vi "Read.vi"(8 "error in (no error)":errorcluster, 11 "SMO.Instrument":refnum<class "SMO.InstrumentDriver.lvclass">) -> (0 "error out":errorcluster, 2 "value":T1, 3 "SMO.Instrument out":refnum<class "SMO.InstrumentDriver.lvclass">)   [LabVIEW 2013, in "SMO.InstrumentDriver.lvclass"]
doc: "---------------------------------------------------------------\nJKI State Machine Objects™\nhttp://jki.net/state-machine-objects/\nCopyright (C) 2005-2015, JKI <info@jki.net>\nALL RIGHTS RESERVEDJKI State Machine Objects (SMO) 1.0.0.5\nJKI - JKI\nCopyright (c) 2016, JKI"
uses:
  SMO.InstrumentDriver.lvclass
  Typedefs/ReadData.ctl
panel:
  # "For instructions on how to use the JKI State Machine Objects, examples and video tutorials, visit:\nhttp://jki.net/state-machine-objects/\n\nJKI State Machine Objects™\nhttp://jki.net/state-machine-objects/\nCopyright (C) 2005-2015, JKI <info@jki.net>\nALL RIGHTS RESERVED"
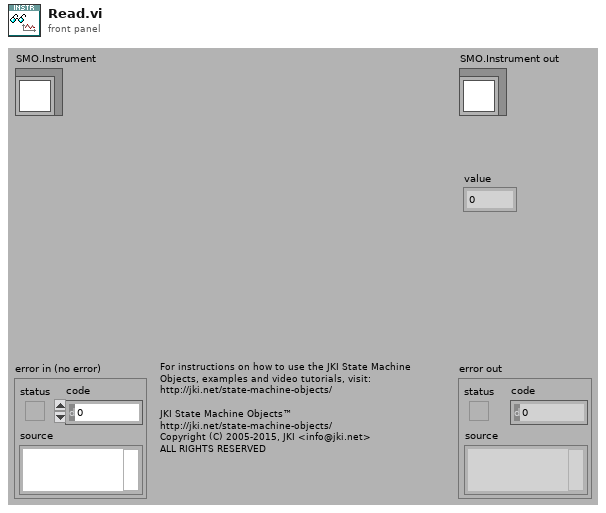
[diagram p1: front panel]
types:
  T1 = typedef "SMO.InstrumentDriver.lvclass/ReadData.ctl" = dbl
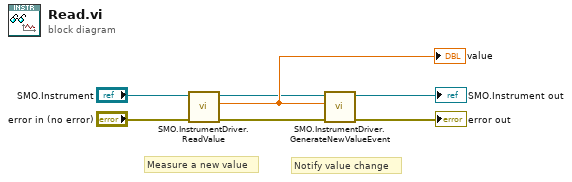
[diagram p0: block diagram]
diagram:
  # "Notify value change"
  # "Measure a new value"
  n1 = call-dynamic "SMO.InstrumentDriver.ReadValue.vi"("error in (no error)"="error in (no error)", "SMO.Instrument"="SMO.Instrument") -> ("error out"=w2:errorcluster, "value"=w5:T1, "SMO.Instrument out"=w4:refnum<class "SMO.InstrumentDriver.lvclass">)  [unwired: 7 in]
  "value" <- w5
  n2 = call "SMO.InstrumentDriver.GenerateNewValueEvent.vi"("error in (no error)"=w2, "value"=w5, "SMO.InstrumentDriver in"=w4) -> ("error out"=→"error out":errorcluster, "SMO.InstrumentDriver out"=→"SMO.Instrument out":refnum<class "SMO.InstrumentDriver.lvclass">)  [unwired: 7 in]
